vi "子VI-深度学习自动检测结果分析.vi"(0 "分层缺陷的面积阈值":i32, 2 "临界Z值":i32, 3 "弥散类缺陷灰度阈值":dbl caption="值", 4 "临界面积百分比值":dbl, 5 "输入的灰度阈值":dbl caption="值", 6 "预测图片保存路径":path, 12 "产品规格":cluster{"产品长度（周长）（mm）":dbl, "产品宽度（母线长）（mm）":dbl}) -> (14 "弥散类检测结果":string[][](table), 16 "全部检测结果":string[][](table), 17 "Threshold Image":T2(plugin-control), 18 "misan":T2(plugin-control))   [LabVIEW 2018]
uses:
  <vilib>/vision/NI_Vision_Development_Module.lvlib
panel:
  out "去掉的面积累计":dbl
  out "?":string[][](table)
  in  "格式字符串 4":string="%f"
  in  "分隔符（'\\'代码显示） 3":string="\t"
  in  "Tab Control":T1
  out "?":T2(plugin-control)
  in  "格式字符串 3":string="%f"
  in  "分隔符（'\\'代码显示） 2":string="\t"
  out "弥散缺陷个数":i32
  out "分层缺陷个数":i32
  out "合格？ 弥散类":string="fencengThreshold"
  out "合格？分层类":string="fencengThreshold"
  out "面积 (pixels)":i32
  in  "格式字符串 2":string="%f"
  in  "分隔符（'\\'代码显示）":string="\t"
  # "所选区域信息"
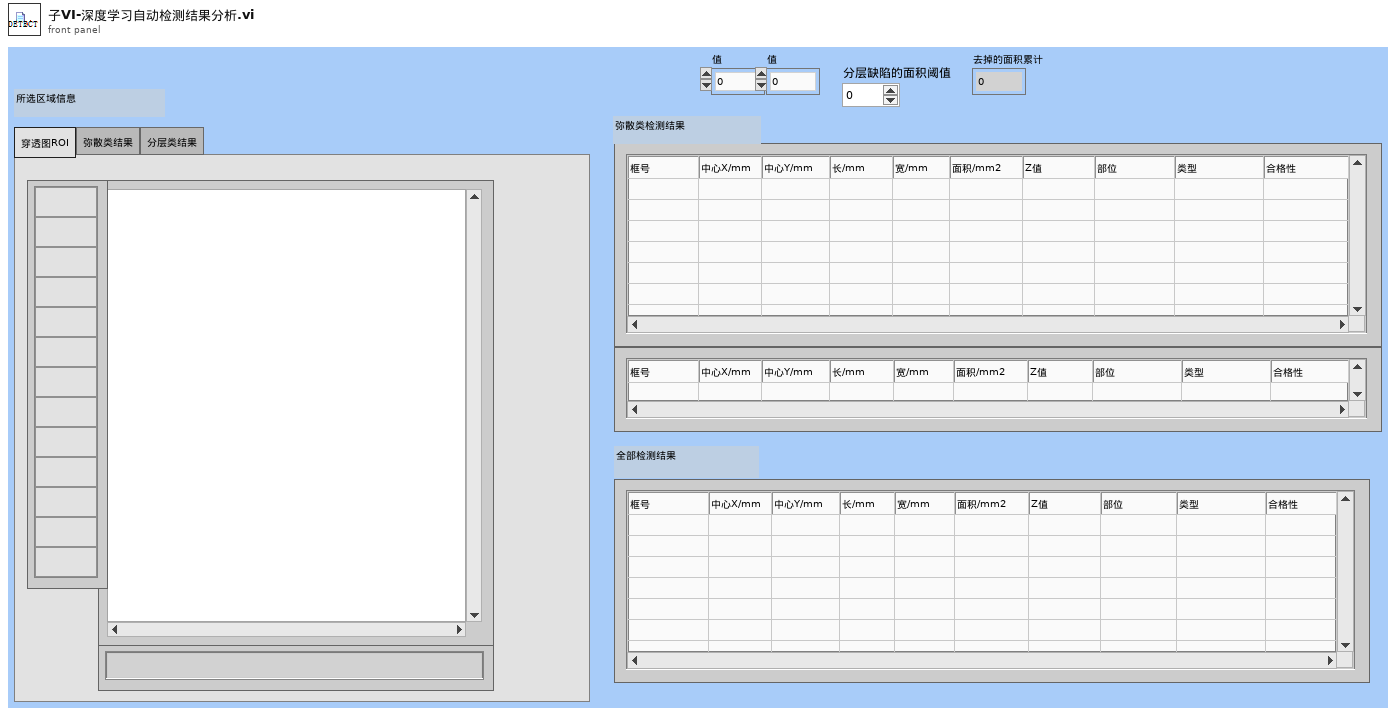
[diagram p1: front panel]
types:
  T1 = typedef "控件2.ctl" = enum32{"穿透图ROI", "弥散类结果", "分层类结果"}
  T2 = typedef "IMAQ Image.ctl" = refnum<image>
  T3 = typedef "Image Type" = u32
  T4 = typedef "Particle Parameters" = i32
  T5 = cluster{"Measurement Parameter":T4, "Range Lower Value":dbl, "Range Upper Value":dbl, "Range":bool, "Measurement Type":bool}[]
  T6 = cluster{"histogram":u32[], "Minimal Value":sgl, "Maximal Value":sgl, "Starting Value":sgl, "Interval Width":sgl, "Mean Value":sgl, "Standard  Variation":sgl, "Area (pixels)":i32}
  T7 = cluster{"Area":dbl, "Number of Holes":dbl, "Bounding Rect":cluster{"Left":dbl, "Top":dbl, "Right":dbl, "Bottom":dbl}, "Center of Mass":cluster{"X":dbl, "Y":dbl}, "Orientation":dbl, "Dimensions":cluster{"Width":dbl, "Height":dbl}}[]
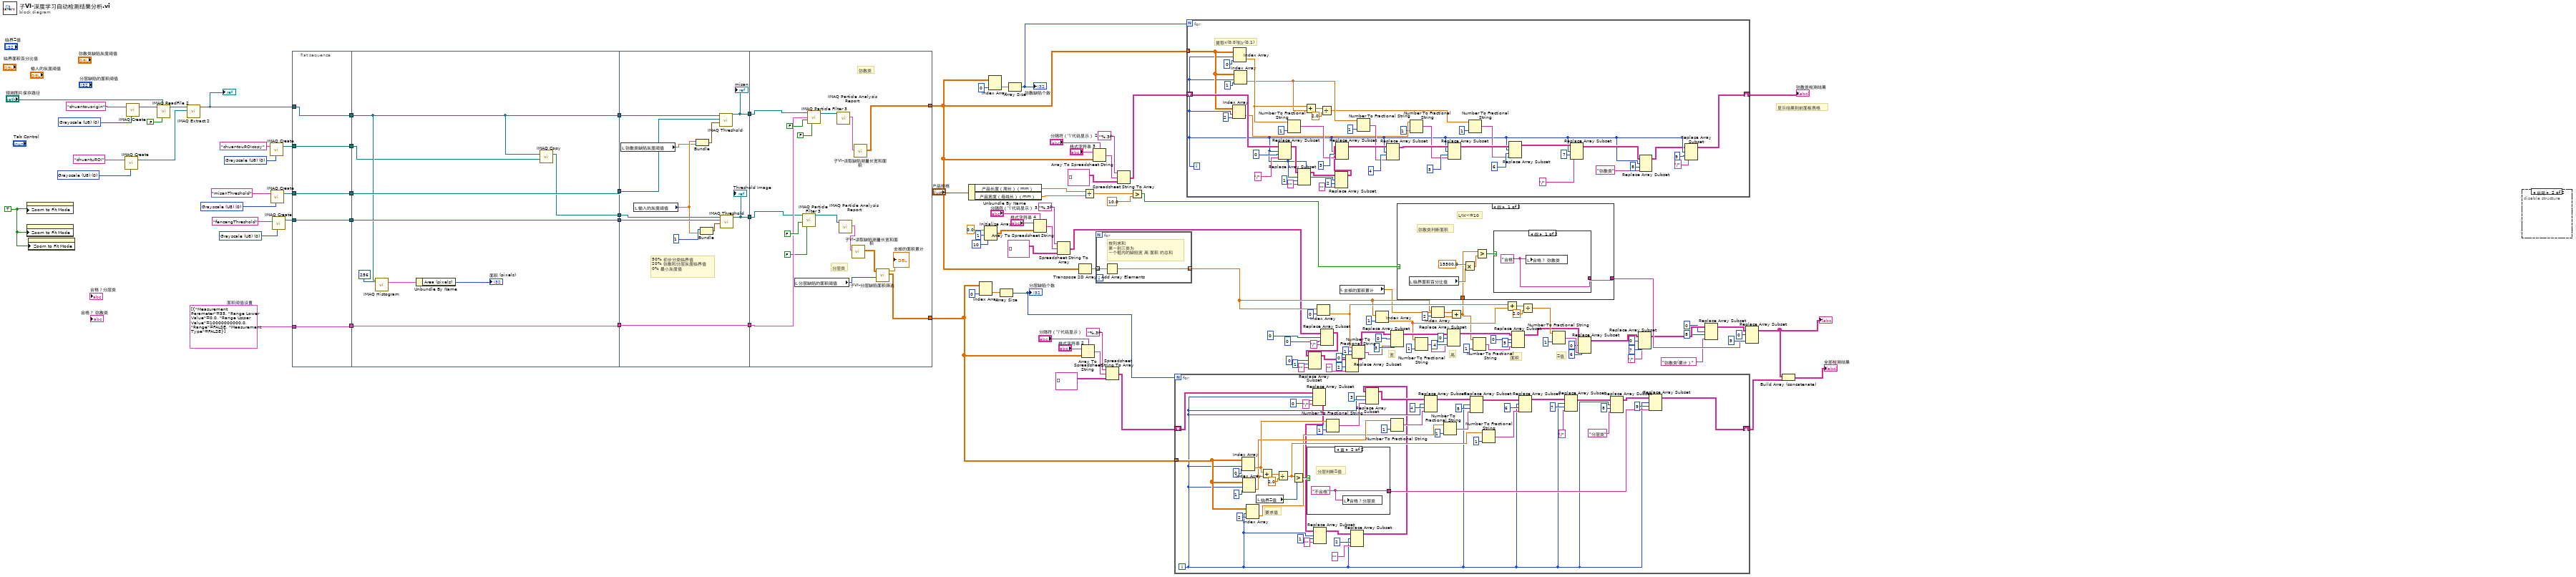
[diagram p0: block diagram]
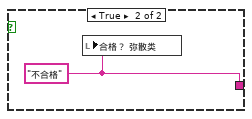
[diagram p2: hidden frame]
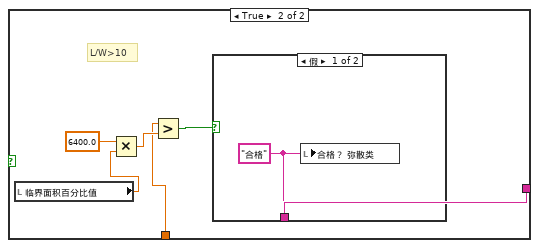
[diagram p3: hidden frame]
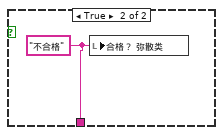
[diagram p4: hidden frame]
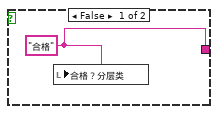
[diagram p5: hidden frame]
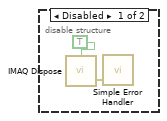
[diagram p6: hidden frame]
diagram:
  w73 = T3 0 items=["Grayscale (U8)", "Grayscale (I16)", "Grayscale (SGL)", "Complex (CSG)", "RGB (U32)", "HSL (U32)", "RGB (U64)", "Grayscale (U16)"] ("Image Type")
  w78 = TRUE ("Zoom to Fit Mode")
  w112 = T3 0 items=["Grayscale (U8)", "Grayscale (I16)", "Grayscale (SGL)", "Complex (CSG)", "RGB (U32)", "HSL (U32)", "RGB (U64)", "Grayscale (U16)"] ("Image Type")
  w113 = T3 0 items=["Grayscale (U8)", "Grayscale (I16)", "Grayscale (SGL)", "Complex (CSG)", "RGB (U32)", "HSL (U32)", "RGB (U64)", "Grayscale (U16)"] ("Image Type")
  w116 = T3 0 items=["Grayscale (U8)", "Grayscale (I16)", "Grayscale (SGL)", "Complex (CSG)", "RGB (U32)", "HSL (U32)", "RGB (U64)", "Grayscale (U16)"] ("Image Type")
  w98 = T5 [{"Measurement Parameter"=35, "Range Lower Value"=0.0, "Range Upper Value"=10000000000.0, "Range"=FALSE, "Measurement Type"=FALSE}]  # 面积阈值设置
  w129 = T3 0 items=["Grayscale (U8)", "Grayscale (I16)", "Grayscale (SGL)", "Complex (CSG)", "RGB (U32)", "HSL (U32)", "RGB (U64)", "Grayscale (U16)"] ("Image Type")
  # "显示结果到前面板表格"
  # "Z值"
  # "面积"
  # "高"
  # "宽"
  n1 = property class="ImageControl"("Zoom to Fit Mode"=w78) -> ()  [unwired: 2 in, 2 out]
  n2 = property class="ImageControl"("Zoom to Fit Mode"=w78) -> ()  [unwired: 2 in, 2 out]
  n3 = property class="ImageControl"("Zoom to Fit Mode"=w78) -> ()  [unwired: 2 in, 2 out]
  n4 = call "IMAQ Create"("Image Name"="chuantuROI", "Image Type"=w116) -> ("New Image"=w115:T2)  [unwired: 3 in, 1 out]
  n5 = call "IMAQ Create"("Image Name"="chuantouorigin", "Image Type"=w129) -> ("New Image"=w118:T2)  [unwired: 3 in, 1 out]
  n6 = call "IMAQ ReadFile 2"("Use File Path Image Type"=FALSE, "File Path"="预测图片保存路径", "Image"=w118) -> ("Image Out"=w119:T2)  [unwired: 4 in, 4 out]
  n7 = call "IMAQ Extract 2"("Image Dst"=w115, "Image Src"=w119) -> ("Image Dst Out"=w81:T2)  [unwired: 8 in, 1 out]
  "?" <- w81
  n8 = call "IMAQ Create"("Image Name"="chuantouROIcopy", "Image Type"=w73) -> ("New Image"=w76:T2)  [unwired: 3 in, 1 out]
  n9 = call "IMAQ Create"("Image Name"="misanThreshold", "Image Type"=w112) -> ("New Image"=w105:T2)  [unwired: 3 in, 1 out]
  n10 = call "IMAQ Create"("Image Name"="fencengThreshold", "Image Type"=w113) -> ("New Image"=w103:T2)  [unwired: 3 in, 1 out]
  n11 = flat-sequence {
    tunnel: w81 -> [w132]
    tunnel: w105 -> [w135]
    tunnel: [w135] -> w106
    tunnel: [w134] -> w104
    tunnel: w103 -> [w134]
    tunnel: [w133] -> w99
    tunnel: w98 -> [w133]
    tunnel: [w132] -> w79
    tunnel: w76 -> [w131]
    tunnel: [w131] -> w75
    tunnel: [w144] -> w107
    tunnel: [w143] -> w102
    tunnel: [w139] -> w97
    tunnel: w99 -> [w139]
    tunnel: w104 -> [w143]
    tunnel: w106 -> [w144]
    tunnel: [w138] -> w80
    tunnel: w79 -> [w138]
    tunnel: [w137] -> w77
    tunnel: w75 -> [w136]
    tunnel: w107 -> [w156]
    tunnel: w102 -> [w155]
    tunnel: [w149] -> w101
    tunnel: [w150] -> w100
    tunnel: w97 -> [w154]
    tunnel: [w154] -> w96
    tunnel: w80 -> [w151]
    tunnel: w77 -> [w148]
    tunnel: [w162] -> w62
    tunnel: [w158] -> w89
    tunnel: w101 -> [w167]
    tunnel: w100 -> [w166]
    tunnel: w96 -> [w170]
    frame #0 {
    }
    frame #1 {
      n12 = call "IMAQ Histogram"("Number of Classes"=256, "Image"=w138) -> ("Histogram Report"=w141:T6)  [unwired: 8 in, 1 out]
      n13 = Unbundle By Name(w141) -> ("Area (pixels)"=→"面积 (pixels)":i32)
      n14 = call "IMAQ Copy"("Image Dst"=w136, "Image Src"=w138) -> ("Image Dst Out"=w137:T2)  [unwired: 4 in, 1 out]
    }
    frame #2 {
      # "50% 初步分类临界值\n20% 弥散和分层灰度临界值\n0% 最小灰度值"
      n15 = local read "弥散类缺陷灰度阈值"() -> (w145:dbl)
      n16 = local read "输入的灰度阈值"() -> (w146:dbl)
      n17 = Bundle("输入的灰度阈值"=w146, "弥散类缺陷灰度阈值"=w145) -> (w153:cluster{"输入的灰度阈值":dbl, "弥散类缺陷灰度阈值":dbl})  [unwired: 1 in]
      n18 = Bundle(1, "输入的灰度阈值"=w146) -> (w152:cluster{i32, "输入的灰度阈值":dbl})  [unwired: 1 in]
      n19 = call "IMAQ Threshold"("Range"=w153, "Image Dst"=w156, "Image Src"=w151) -> ("Image Dst Out"=w150:T2)  [unwired: 3 in, 5 out]
      "misan" <- w150
      n20 = call "IMAQ Threshold"("Range"=w152, "Image Dst"=w155, "Image Src"=w148) -> ("Image Dst Out"=w149:T2)  [unwired: 3 in, 5 out]
      "Threshold Image" <- w149
    }
    frame #3 {
      # "分层类"
      # "弥散类"
      n21 = local read "分层缺陷的面积阈值"() -> (w159:i32)
      n22 = call "IMAQ Particle Filter 3"("Image Src"=w167, "Keep/Remove Particles (F)"=FALSE, "Reject Border? (F)"=FALSE) -> ("Image Dst Out"=w165:T2)  [unwired: 10 in, 2 out]
      n23 = call "IMAQ Particle Filter 3"("Image Src"=w166, "Selection Values"=w170, "Keep/Remove Particles (F)"=FALSE, "Reject Border? (F)"=FALSE) -> ("Image Dst Out"=w161:T2)  [unwired: 9 in, 2 out]
      n24 = call "IMAQ Particle Analysis Report"("Image"=w161) -> ("Particle Reports (Pixels)"=w163:T7)  [unwired: 5 in, 5 out]
      n25 = call "IMAQ Particle Analysis Report"("Image"=w165) -> ("Particle Reports (Pixels)"=w164:T7)  [unwired: 5 in, 5 out]
      n26 = call "子VI-读取缺陷测量长宽和面积.vi"("Particle Reports (Pixels)"=w164) -> ("测量结果"=w160:dbl[][])  [unwired: 10 in]
      n27 = call "子VI-读取缺陷测量长宽和面积.vi"("Particle Reports (Pixels)"=w163) -> ("测量结果"=w162:dbl[][])  [unwired: 10 in]
      n28 = call "子VI-分层缺陷面积筛选.vi"("计入分层缺陷的面积阈值"=w159, "分层测量结果"=w160) -> ("初始化的数组"=w158:dbl[][], "去掉的面积累计"=→"去掉的面积累计":dbl)  [unwired: 8 in]
    }
  }
  n29 = Unbundle By Name("产品规格") -> ("产品长度（周长）（mm）"=w123:dbl, "产品宽度（母线长）（mm）"=w122:dbl)
  n30 = Index Array(array=w89, index (col)=0 ("禁用的索引 (列)")) -> (element=w111:dbl[])  [unwired: 1 in]
  n31 = Initialize Array(0.0 ("元素"), 1 ("维数大小"), 10 ("维数大小")) -> (w63:dbl[][])
  n32 = Index Array(array=w62, index (col)=0 ("禁用的索引 (列)")) -> (element=w109:dbl[])  [unwired: 1 in]
  n33 = Array Size(array=w111) -> (size(s)=w95:i32)
  "分层缺陷个数" <- w95
  n34 = Array Size(array=w109) -> (size(s)=w121:i32)
  "弥散缺陷个数" <- w121
  n35 = Array To Spreadsheet String(delimiter (Tab)="分隔符（'\\'代码显示） 3", array=w63, 3:"格式字符串 4") -> (spreadsheet string=w66:string)
  n36 = Spreadsheet String To Array(format string="%.3f", spreadsheet string=w66, array type (2D Dbl)=string[][] [] ("Array")) -> (array=w40:string[][])  [unwired: 1 in]
  n37 = Transpose 2D Array(2D array=w62) -> (transposed array=w72:dbl[][])
  n38 = Array To Spreadsheet String(delimiter (Tab)="分隔符（'\\'代码显示）", array=w89, 3:"格式字符串 2") -> (spreadsheet string=w92:string)
  n39 = Divide(x=w123, y=w122) -> (x/y=w126:dbl)
  n40 = Array To Spreadsheet String(delimiter (Tab)="分隔符（'\\'代码显示） 2", array=w62, 3:"格式字符串 3") -> (spreadsheet string=w85:string)
  n41 = for {
    tunnel: w72 -> [w174] mode=indexing
    tunnel: [w173] -> w41 mode=indexing
    # "按列求和 \n第一到三类为\n一个框内的缺陷宽 高 面积 的总和"
    n42 = Add Array Elements(numeric array=w174) -> (sum=w173:dbl)
  }
  n43 = Spreadsheet String To Array(format string="%.3f", spreadsheet string=w92, array type (2D Dbl)=string[][] [] ("Array")) -> (array=w88:string[][])  [unwired: 1 in]
  n44 = Spreadsheet String To Array(format string="%.3f", spreadsheet string=w85, array type (2D Dbl)=string[][] [] ("Array")) -> (array=w82:string[][])  [unwired: 1 in]
  n45 = Greater?(x=w126, y=10.0) -> (0:w39:bool)
  n46 = for {
    N: w95 -> [_]
    tunnel: w89 -> [w194]
    shift-right: [w201] -> w26
    shift-left: w88 -> [w209]
    i -> [w182]
    # "要求值"
    n47 = Index Array(array=w194, index (row)=w182, index (col)=0 ("禁用的索引 (列)")) -> (element=w200:dbl)
    n48 = Index Array(array=w194, index (row)=w182, index (col)=1 ("禁用的索引 (列)")) -> (element=w199:dbl)
    n49 = Index Array(array=w194, index (row)=w182, index (col)=2 ("禁用的索引 (列)")) -> (element=w192:dbl)
    n50 = local read "临界Z值"() -> (w220:i32)
    n51 = Add(x=w200, y=w199) -> (x+y=w221:dbl)
    n52 = Divide(x=w221, y=2.0) -> (x/y=w197:dbl)
    n53 = Greater?(x=w197, y=w220) -> (0:w222:bool)
    n54 = case shown="真" w222 {
      tunnel: [w223 w224] -> w196
      frame False {
        w223 = "合格" ("合格？")
        n55 = local write "合格？分层类"(w223) -> ()
      }
      frame True {
        w224 = "不合格" ("合格？")
        # "分层判断Z值"
        n56 = local write "合格？分层类"(w224) -> ()
      }
    }
    n57 = Replace Array Subset(array=w209, new element="/" ("新元素/子数组"), index (row)=w182, index (col)=0 ("索引 (列)")) -> (w180:string[][])
    n58 = Replace Array Subset(array=w180, new element="" ("新元素/子数组"), index (row)=w182, index (col)=1 ("索引 (列)")) -> (w189:string[][])
    n59 = Number To Fractional String(number=w200, precision (6)=i16 1 ("精度(6)")) -> (F-format string=w208:string)  [unwired: 2 in]
    n60 = Replace Array Subset(array=w189, new element="" ("新元素/子数组"), index (row)=w182, index (col)=2 ("索引 (列)")) -> (w179:string[][])
    n61 = Replace Array Subset(array=w179, new element=w208, index (row)=w182, index (col)=3 ("索引 (列)")) -> (w206:string[][])
    n62 = Number To Fractional String(number=w199, precision (6)=i16 1 ("精度(6)")) -> (F-format string=w207:string)  [unwired: 2 in]
    n63 = Replace Array Subset(array=w206, new element=w207, index (row)=w182, index (col)=4 ("索引 (列)")) -> (w205:string[][])
    n64 = Number To Fractional String(number=w192, precision (6)=i16 1 ("精度(6)")) -> (F-format string=w204:string)  [unwired: 2 in]
    n65 = Replace Array Subset(array=w205, new element=w204, index (row)=w182, index (col)=5 ("索引 (列)")) -> (w203:string[][])
    n66 = Number To Fractional String(number=w197, precision (6)=i16 1 ("精度(6)")) -> (F-format string=w198:string)  [unwired: 2 in]
    n67 = Replace Array Subset(array=w203, new element=w198, index (row)=w182, index (col)=6 ("索引 (列)")) -> (w202:string[][])
    n68 = Replace Array Subset(array=w202, new element="/" ("新元素/子数组"), index (row)=w182, index (col)=7 ("索引 (列)")) -> (w185:string[][])
    n69 = Replace Array Subset(array=w185, new element="分层类" ("新元素/子数组"), index (row)=w182, index (col)=8 ("禁用的索引 (列)")) -> (w183:string[][])
    n70 = Replace Array Subset(array=w183, new element=w196, index (row)=w182, index (col)=9 ("索引 (列)")) -> (w201:string[][])
  }
  n71 = for {
    N: w121 -> [_]
    tunnel: w62 -> [w243]
    shift-right: [w256] -> w19
    shift-left: w82 -> [w261]
    i -> [w226]
    # "提取x(0,0)和y(0,1)"
    n72 = Index Array(array=w243, index (row)=w226, index (col)=2 ("索引 (列)")) -> (element=w242:dbl)
    n73 = Index Array(array=w243, index (row)=w226, index (col)=0 ("禁用的索引 (列)")) -> (element=w250:dbl)
    n74 = Index Array(array=w243, index (row)=w226, index (col)=1 ("禁用的索引 (列)")) -> (element=w249:dbl)
    n75 = Replace Array Subset(array=w261, new element="/" ("新元素/子数组"), index (row)=w226, index (col)=0 ("索引 (列)")) -> (w238:string[][])
    n76 = Number To Fractional String(number=w250, precision (6)=i16 1 ("精度(6)")) -> (F-format string=w255:string)  [unwired: 2 in]
    n77 = Replace Array Subset(array=w238, new element="" ("新元素/子数组"), index (row)=w226, index (col)=1 ("索引 (列)")) -> (w237:string[][])
    n78 = Add(x=w250, y=w249) -> (x+y=w252:dbl)
    n79 = Divide(x=w252, y=2.0) -> (x/y=w248:dbl)
    n80 = Replace Array Subset(array=w237, new element="" ("新元素/子数组"), index (row)=w226, index (col)=2 ("索引 (列)")) -> (w236:string[][])
    n81 = Replace Array Subset(array=w236, new element=w255, index (row)=w226, index (col)=3 ("索引 (列)")) -> (w260:string[][])
    n82 = Number To Fractional String(number=w249, precision (6)=i16 1 ("精度(6)")) -> (F-format string=w254:string)  [unwired: 2 in]
    n83 = Replace Array Subset(array=w260, new element=w254, index (row)=w226, index (col)=4 ("索引 (列)")) -> (w259:string[][])
    n84 = Number To Fractional String(number=w242, precision (6)=i16 1 ("精度(6)")) -> (F-format string=w253:string)  [unwired: 2 in]
    n85 = Replace Array Subset(array=w259, new element=w253, index (row)=w226, index (col)=5 ("索引 (列)")) -> (w258:string[][])
    n86 = Number To Fractional String(number=w248, precision (6)=i16 1 ("精度(6)")) -> (F-format string=w247:string)  [unwired: 2 in]
    n87 = Replace Array Subset(array=w258, new element=w247, index (row)=w226, index (col)=6 ("索引 (列)")) -> (w257:string[][])
    n88 = Replace Array Subset(array=w257, new element="/" ("新元素/子数组"), index (row)=w226, index (col)=7 ("索引 (列)")) -> (w229:string[][])
    n89 = Replace Array Subset(array=w229, new element="弥散类" ("新元素/子数组"), index (row)=w226, index (col)=8 ("禁用的索引 (列)")) -> (w225:string[][])
    n90 = Replace Array Subset(array=w225, new element="/" ("新元素/子数组"), index (row)=w226, index (col)=9 ("索引 (列)")) -> (w256:string[][])
  }
  "弥散类检测结果" <- w19
  n91 = Index Array(array=w41, index=0 ("索引")) -> (element=w43:dbl)
  n92 = Replace Array Subset(array=w40, new element="/" ("新元素/子数组"), index (row)=0 ("禁用的索引 (行)"), index (col)=0 ("索引 (列)")) -> (w18:string[][])
  n93 = Replace Array Subset(array=w18, new element="" ("新元素/子数组"), index (row)=0 ("禁用的索引 (行)"), index (col)=1 ("索引 (列)")) -> (w23:string[][])
  n94 = local read "去掉的面积累计"() -> (w2:dbl)
  n95 = Replace Array Subset(array=w23, new element="" ("新元素/子数组"), index (row)=0 ("禁用的索引 (行)"), index (col)=2 ("索引 (列)")) -> (w17:string[][])
  n96 = Number To Fractional String(number=w43, precision (6)=i16 1 ("精度(6)")) -> (F-format string=w56:string)  [unwired: 2 in]
  n97 = Index Array(array=w41, index=1 ("索引")) -> (element=w42:dbl)
  n98 = Replace Array Subset(array=w17, new element=w56, index (row)=0 ("索引 (行)"), index (col)=3 ("索引 (列)")) -> (w54:string[][])
  n99 = Number To Fractional String(number=w42, precision (6)=i16 1 ("精度(6)")) -> (F-format string=w47:string)  [unwired: 2 in]
  n100 = Index Array(array=w41, index=2 ("索引")) -> (element=w3:dbl)
  n101 = Replace Array Subset(array=w54, new element=w47, index (row)=0 ("索引 (行)"), index (col)=4 ("禁用的索引 (列)")) -> (w49:string[][])
  n102 = Add(x=w2, y=w3) -> (x+y=w1:dbl)
  n103 = case shown="假" w39 {
    tunnel: [w275 w283] -> w27
    tunnel: w1 -> [w271 w279]
    frame False {
      # "弥散类判断面积"
      # "L/W<=10"
      n104 = local read "临界面积百分比值"() -> (w273:dbl)
      n105 = Multiply(x=15500.0, y=w273) -> (x*y=w272:dbl)
      n106 = Greater?(x=w271, y=w272) -> (0:w276:bool)
      n107 = case shown="假" w276 {
        tunnel: [w277 w278] -> w275
        frame False {
          w277 = "合格" ("合格？")
          n108 = local write "合格？ 弥散类"(w277) -> ()
        }
        frame True {
          w278 = "不合格" ("合格？")
          n109 = local write "合格？ 弥散类"(w278) -> ()
        }
      }
    }
    frame True {
      # "L/W>10"
      n110 = local read "临界面积百分比值"() -> (w280:dbl)
      n111 = Multiply(x=6400.0, y=w280) -> (x*y=w282:dbl)
      n112 = Greater?(x=w279, y=w282) -> (0:w284:bool)
      n113 = case shown="假" w284 {
        tunnel: [w285 w286] -> w283
        frame False {
          w285 = "合格" ("合格？")
          n114 = local write "合格？ 弥散类"(w285) -> ()
        }
        frame True {
          w286 = "不合格" ("合格？")
          n115 = local write "合格？ 弥散类"(w286) -> ()
        }
      }
    }
  }
  n116 = Number To Fractional String(number=w1, precision (6)=i16 1 ("精度(6)")) -> (F-format string=w46:string)  [unwired: 2 in]
  n117 = Add(x=w43, y=w42) -> (x+y=w45:dbl)
  n118 = Replace Array Subset(array=w49, new element=w46, index (row)=0 ("索引 (行)"), index (col)=5 ("索引 (列)")) -> (w34:string[][])
  n119 = Divide(x=w45, y=2.0) -> (x/y=w35:dbl)
  n120 = Number To Fractional String(number=w35, precision (6)=i16 1 ("精度(6)")) -> (F-format string=w38:string)  [unwired: 2 in]
  n121 = Replace Array Subset(array=w34, new element=w38, index (row)=0 ("索引 (行)"), index (col)=6 ("索引 (列)")) -> (w31:string[][])
  n122 = Replace Array Subset(array=w31, new element="/" ("新元素/子数组"), index (row)=0 ("索引 (行)"), index (col)=7 ("索引 (列)")) -> (w12:string[][])
  n123 = Replace Array Subset(array=w12, new element="弥散类(累计）" ("新元素/子数组"), index (row)=0 ("索引 (行)"), index (col)=8 ("禁用的索引 (列)")) -> (w8:string[][])
  n124 = Replace Array Subset(array=w8, new element=w27, index (row)=0 ("索引 (行)"), index (col)=9 ("索引 (列)")) -> (w21:string[][])
  "?" <- w21
  n125 = Build Array (concatenate)(w21, w26) -> (→"全部检测结果":string[][])
  n126 = disable-structure shown="启用" {
    frame Disabled {
      n127 = call "IMAQ Dispose"("All Images? (No)"=TRUE) -> ("error out"=w288:errorcluster)  [unwired: 5 in]
      n128 = call <vilib>:"Simple Error Handler.vi"("error in (no error)"=w288) -> ()  [unwired: 4 in, 5 out]
    }
    frame Enabled {
    }
  }
